vi "标定.vi"(7 "error in":errorcluster) -> (27 "error out":errorcluster)   [LabVIEW 2014]
uses:
  <vilib>/vision/Image Controls.llb/Vision Info Type2.ctl
  <vilib>/vision/NI_Vision_Development_Module.lvlib
panel:
  out "Image Out":T1(plugin-control)
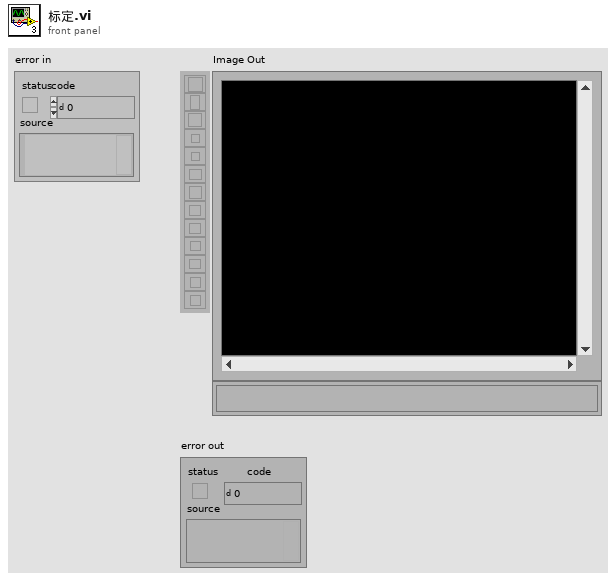
[diagram p1: front panel]
types:
  T1 = typedef "IMAQ Image.ctl" = refnum<image>
  T2 = cluster{"Origin Pixel":cluster{"X":sgl, "Y":sgl}, "X Axis Pixel":cluster{"X":sgl, "Y":sgl}, "Axis Reference":u32}
  T3 = typedef "Vision Info Type2.ctl" = u32
  T4 = typedef "Simple Grid Descriptor" = cluster{"X Step":sgl, "Y Step":sgl, "Unit":T5}
  T5 = typedef "Image Unit" = enum32{"Undefined", "Angström", "Micrometer", "Millimeter", "Centimeter", "Meter", "Kilometer", "Microinch", "Inch", "Feet", "Nautical miles", "Standard miles", "Steps"}
  T6 = typedef "Image Type" = u32
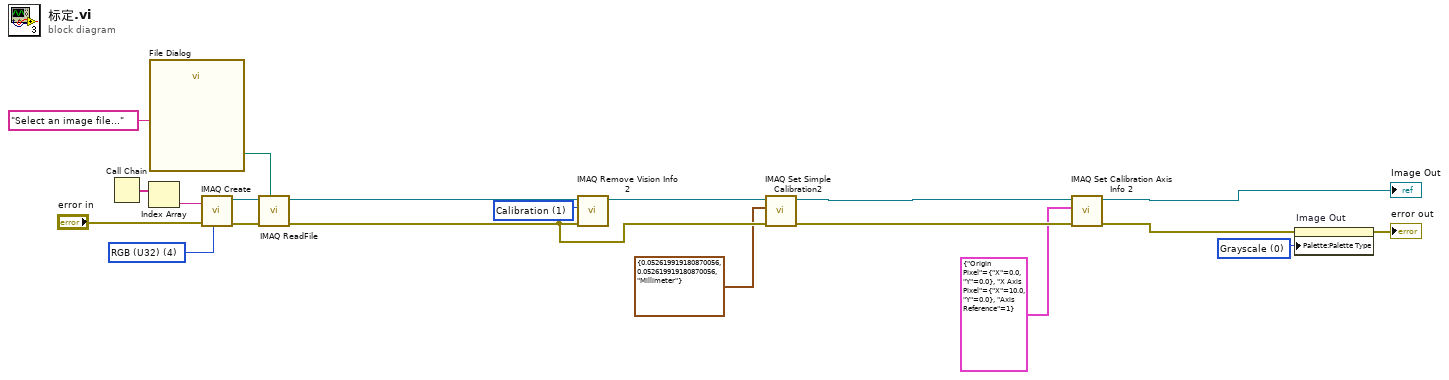
[diagram p0: block diagram]
diagram:
  w1 = u32 0 items=["Grayscale", "Binary", "Gradient", "Rainbow", "Temperature", "User Defined", "Binary 16 Bit", "Gradient 16 Bit", "Rainbow 16 Bit", "Temperature 16 Bit", "User Defined 16 Bit"] ("Palette Type")
  w10 = T3 1 items=["Any", "Calibration", "Overlay", "Grayscale Template", "Color Template", "Geometric Template", "Custom Data", "Golden Template", "Geometric Template 2", "Contour Data", "Camera Model"] ("Vision Info")
  w12 = T6 4 items=["Grayscale (U8)", "Grayscale (I16)", "Grayscale (SGL)", "Complex (CSG)", "RGB (U32)", "HSL (U32)", "RGB (U64)", "Grayscale (U16)"] ("Image Type")
  n1 = Call Chain() -> (call chain=w16:string[])
  n2 = Index Array(array=w16) -> (element=w15:string)  [unwired: 1 in]
  n3 = call "File Dialog"("prompt"="Select an image file...") -> ("selected path"=w13:path)  [unwired: 6 in, 8 out]
  n4 = call "IMAQ Create"("Image Name"=w15, "Image Type"=w12, "error in (no error)"="error in") -> ("New Image"=w19:T1, "error out"=w18:errorcluster)  [unwired: 1 in, 1 out]
  n5 = call "IMAQ ReadFile"("File Path"=w13, "error in (no error)"=w18, "Image"=w19) -> ("error out"=w20:errorcluster, "Image Out"=w9:T1)  [unwired: 2 in, 5 out]
  n6 = call "IMAQ Remove Vision Info 2"("error in (no error)"=w20, "Vision Info"=w10, "Image"=w9) -> ("Image Out"=w8:T1)  [unwired: 8 out]
  n7 = call "IMAQ Set Simple Calibration2"("error in (no error)"=w20, "Pixel Distances"=T4 {"X Step"=0.05261992, "Y Step"=0.05261992, "Unit"=enum."Millimeter"} ("Grid Descriptor"), "Image"=w8) -> ("error out"=w7:errorcluster, "Calibration Template Image"=w5:T1)  [unwired: 2 in, 5 out]
  n8 = call-poly "IMAQ Set Calibration Axis Info 2"("error in (no error)"=w7, "Calibration Axis Info"=T2 {"Origin Pixel"={"X"=0.0, "Y"=0.0}, "X Axis Pixel"={"X"=10.0, "Y"=0.0}, "Axis Reference"=1}, "Calibration Template Image In"=w5) -> ("error out"=w6:errorcluster, "Calibration Template Image Out"=→"Image Out":T1)  [unwired: 7 out]
  n9 = property on="Image Out" class="ImageControl"(error in=w6, "Palette:Palette Type"=w1) -> (error out=→"error out":errorcluster)  [unwired: 1 in, 1 out]
